vi "Excercise 3-5.vi"() -> ()   [LabVIEW 2014]
panel:
  out "Warning?":bool
  out "Warning Text":string
  in  "Min Temp":dbl
  in  "Max Temp":dbl
  in  "Current Temp":dbl
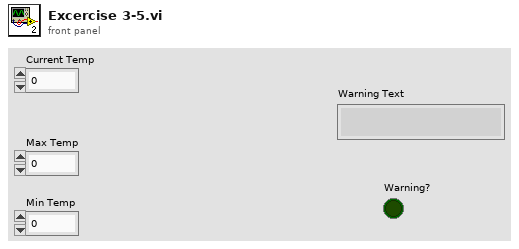
[diagram p1: front panel]
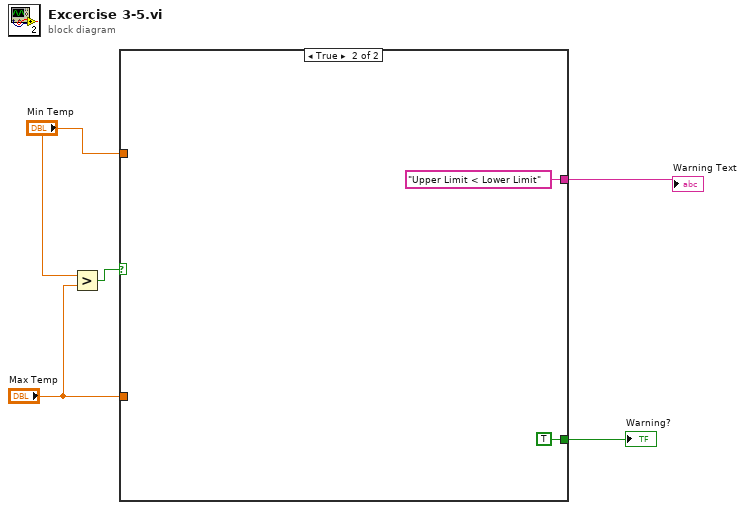
[diagram p0: block diagram]
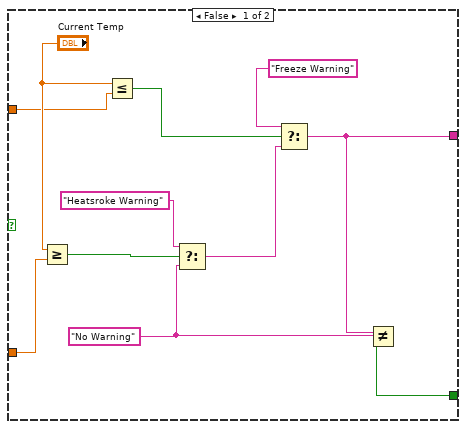
[diagram p2: hidden frame]
diagram:
  n1 = Greater?(x="Min Temp", y="Max Temp") -> (0:w1:bool)
  n2 = case shown="True" w1 {
    tunnel: [w9 TRUE] -> w5
    tunnel: [w8 "Upper Limit < Lower Limit"] -> w4
    tunnel: "Min Temp" -> [w7 _]
    tunnel: "Max Temp" -> [w6 _]
    frame False {
      w10 = "No Warning"
      n3 = Greater Or Equal?(x="Current Temp", y=w6) -> (x >= y?=w15:bool)
      n4 = Less Or Equal?(x="Current Temp", y=w7) -> (x <= y?=w13:bool)
      n5 = Select(t="Heatsroke Warning", s=w15, f=w10) -> (s? t:f=w11:string)
      n6 = Select(t="Freeze Warning", s=w13, f=w11) -> (s? t:f=w8:string)
      n7 = Not Equal?(x=w8, y=w10) -> (x != y?=w9:bool)
    }
    frame True {
    }
  }
  "Warning Text" <- w4
  "Warning?" <- w5
